vi "time pressed.vi"(11 "NXT":T2={"error"={"status"=FALSE, "code"=0, "source"=""}, "address"="", "NXT #"=0, "Show Error"=FALSE, "Connection"=4} {"Connection" items=["USB", "Bluetooth", "USB then Bluetooth", "Last Connection", "Preference"]}) -> (1 "time pressed (ms)":u32, 2 "Buttons pressed":T1 items=["None", "Center", "Left", "C+L", "Right", "C+R", "C+L", "All"], 3 "NXT 2":T2={"error"={"status"=FALSE, "code"=0, "source"=""}, "address"="", "NXT #"=-1, "Show Error"=TRUE, "Connection"=4} {"Connection" items=["USB", "Bluetooth", "USB then Bluetooth", "Last Connection", "Preference"]})   [LabVIEW 2009]
doc: "\"time pressed\" is the time the buttons have been\nheld down in this configuration.\n\nButton Pressed Values:\n0 - None\n1 - Center\n2 - Left\n3 - Center + Left\n4 - Right\n5 - Center + Right\n6 - Left + Right\n7 - All"
uses:
  <vilib>/NXT/Subs/LVHSConnector.ctl
  buttons pressed.ctl
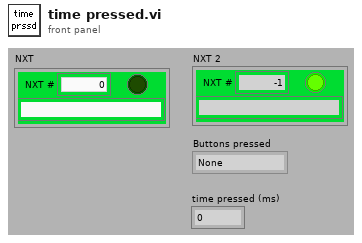
[diagram p1: front panel]
types:
  T1 = typedef "buttons pressed.ctl" = u8
  T2 = typedef "LVHSConnector.ctl" = cluster{"error":errorcluster, "address":string, "NXT #":i32, "Show Error":bool, "Connection":u16}
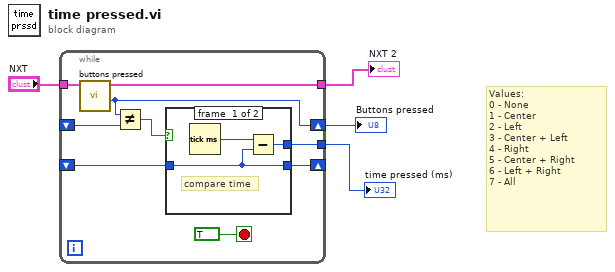
[diagram p0: block diagram]
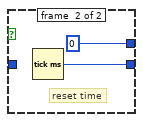
[diagram p2: hidden frame]
diagram:
  # "Values:\n0 - None\n1 - Center\n2 - Left\n3 - Center + Left\n4 - Right\n5 - Center + Right\n6 - Left + Right\n7 - All"
  n1 = while {
    tunnel: "NXT" -> [w13]
    tunnel: [w12] -> w3
    shift-right: [w10] -> w2
    shift-left: _ -> [w9]
    shift-right: [w7] -> _
    shift-left: _ -> [w5]
    tunnel: [w6] -> w1
    stop <- TRUE stop-if-true
    n2 = call "buttons pressed.vi"("NXT 2"=w13) -> ("Buttons pressed"=w10:T1, "NXT"=w12:T2)  [unwired: 9 in]
    n3 = Not Equal?(x=w10, y=w9) -> (x != y?=w8:bool)
    n4 = case shown="False" w8 {
      tunnel: [w14 w18] -> w7
      tunnel: [w15 u32 0 ("time pressed (ms)")] -> w6
      tunnel: w5 -> [w14 _]
      frame #0 {
        # "compare time"
        n5 = Tick Count (ms)() -> (millisecond timer value=w16:u32)
        n6 = Subtract(x=w16, y=w14) -> (x-y=w15:u32)
      }
      frame #1 {
        # "reset time"
        n7 = Tick Count (ms)() -> (millisecond timer value=w18:u32)
      }
    }
  }
  "NXT 2" <- w3
  "Buttons pressed" <- w2
  "time pressed (ms)" <- w1
